vi "Quit.vi"(8 "error in (no error)":errorcluster, 11 "Engine in":refnum<class "Engine.lvclass">) -> (0 "error out":errorcluster)   [LabVIEW 2024, in "GLF.lvlib" / "Engine.lvclass"]
uses:
  Engine.lvclass
  Engine.lvclass/Engine.ctl
  Command--enum.ctl
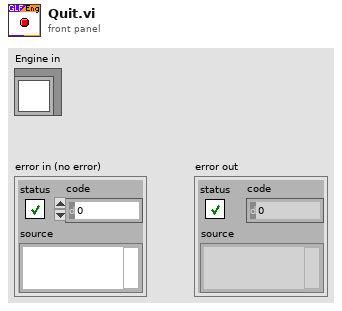
[diagram p1: front panel]
types:
  T1 = typedef "GLF.lvlib/Engine.lvclass/Command--enum.ctl" = enum16{"Quit", "Register Window"}
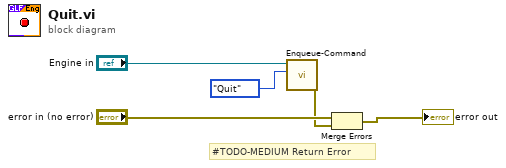
[diagram p0: block diagram]
diagram:
  # "#TODO-MEDIUM Return Error"
  n1 = call "Enqueue-Command.vi"("Cmd"=Command--enum."Quit", "Engine in"="Engine in") -> ("error out"=w1:errorcluster)  [unwired: 7 in, 2 out]
  n2 = Merge Errors("error in (no error)", w1) -> (→"error out":errorcluster)
